vi "Gesture Handler.vi"(9 "gesture":refnum<class "Gesture.lvclass">, 10 "tracking in":bool, 11 "Blob in":refnum<class "Blob.lvclass">) -> (1 "stop?":bool, 2 "tracking out":bool, 3 "Blob out":refnum<class "Blob.lvclass">)   [LabVIEW 2019, in "Blob.lvclass"]
doc: "Given the current tracking state, and the current gesture, manipulate the Blob object appropriately."
uses:
  Blob.lvclass
  Gesture/Gesture.lvclass
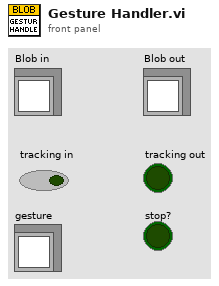
[diagram p1: front panel]
types:
  T1 = typedef "LVPoint32TypeDef.ctl" = cluster{"Horizontal":i32, "Vertical":i32}
  T2 = typedef "Gesture.lvclass/Gesture Enum.ctl" = enum16{"None", "Stop", "Tap", "Press", "Pan Start", "Pan Continue", "Pan End", "Pinch Open", "Pinch Close", "Double Tap"}
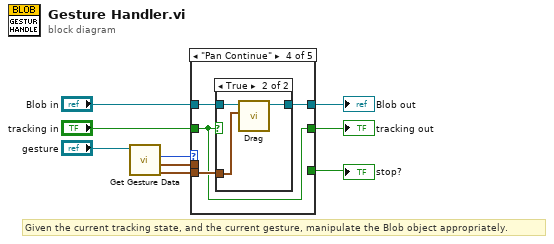
[diagram p0: block diagram]
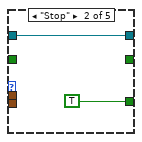
[diagram p3: hidden frame]
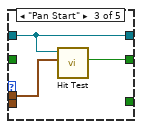
[diagram p4: hidden frame]
diagram:
  # "Given the current tracking state, and the current gesture, manipulate the Blob object appropriately."
  n1 = call-dynamic "Get Gesture Data.vi"("gesture in"="gesture") -> ("offset"=w2:T1, "point"=w5:T1, "gesture"=w8:T2)  [unwired: 6 in, 2 out]
  n2 = case shown="\"Pan Continue\"" w8 {
    tunnel: [w10 w12 w13 w18 w24] -> w7
    tunnel: "Blob in" -> [w10 w12 w13 w19 w24]
    tunnel: w5 -> [_ _ w15 _ _]
    tunnel: [_ _ w14 w16 _] -> w4
    tunnel: "tracking in" -> [_ _ _ w16 _]
    tunnel: w2 -> [_ _ _ w17 _]
    tunnel: [_ TRUE _ _ _] -> w1
    frame Default {
    }
    frame "Stop" {
    }
    frame "Pan Start" {
      n3 = call-dynamic "Hit Test.vi"("point"=w15, "Blob in"=w13) -> ("hit"=w14:bool)  [unwired: 9 in]
    }
    frame "Pan Continue" {
      n4 = case shown="True" w16 {
        tunnel: w19 -> [w20 w23]
        tunnel: [w20 w22] -> w18
        tunnel: w17 -> [_ w21]
        frame False {
        }
        frame True {
          n5 = call-dynamic "Drag.vi"("offset"=w21, "Blob in"=w23) -> ("Blob out"=w22:refnum<class "Blob.lvclass">)  [unwired: 9 in]
        }
      }
    }
    frame "Pan End" {
    }
  }
  "Blob out" <- w7
  "tracking out" <- w4
  "stop?" <- w1
